vi "CreateOrAddLibraryToProject.vi"(8 "error in (no error)":errorcluster, 10 "Library Path In (Create New)":path, 11 "Project Reference In (Create New)":refnum<vi>) -> (0 "error out":errorcluster, 2 "Library Reference Out":refnum<vi>, 3 "Project Reference Out":refnum<vi>)   [LabVIEW 2017]
doc: "Creates a new library or opens an existing one and adds it to a project or to a new project."
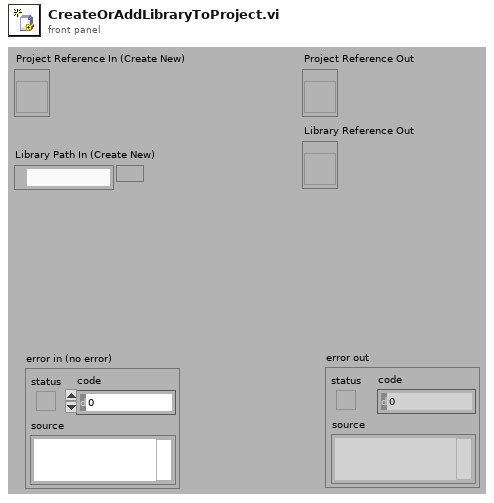
[diagram p1: front panel]
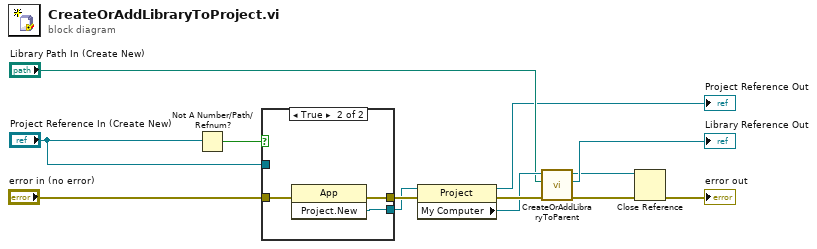
[diagram p0: block diagram]
diagram:
  n1 = Not A Number/Path/Refnum?(number/path/refnum="Project Reference In (Create New)") -> (NaN/Path/Refnum?=w13:bool)
  n2 = case shown="True" w13 {
    tunnel: "Project Reference In (Create New)" -> [w15 _]
    tunnel: [w15 w18] -> w9
    tunnel: "error in (no error)" -> [w14 w17]
    tunnel: [w14 w16] -> w10
    frame False {
    }
    frame True {
      n3 = invoke class="App" method="Project.New"(error in=w17) -> (error out=w16:errorcluster, "Project:New"=w18:refnum<vi>)  [unwired: 2 in, 1 out]
    }
  }
  n4 = property class="Project"(reference=w9, error in=w10) -> (reference out=→"Project Reference Out":refnum<vi>, error out=w8:errorcluster, "My Computer"=w7:refnum<vi>)
  n5 = call <vilib>:"CreateOrAddLibraryToParent.vi"("error in (no error)"=w8, "Library Path In (Create New)"="Library Path In (Create New)", "Parent Reference In"=w7) -> ("error out"=w3:errorcluster, "Library Reference Out"=→"Library Reference Out":refnum<vi>, "Parent Reference Out"=w2:refnum<vi>)  [unwired: 6 in]
  n6 = Close Reference(reference=w2, error in (no error)=w3) -> (error out=→"error out":errorcluster)
